vi "Round_Three_Decimals.vi"(11 "Number Input":dbl) -> (3 "Number Output":dbl)   [LabVIEW 2020]
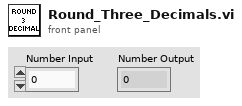
[diagram p1: front panel]
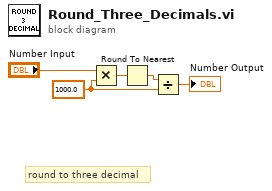
[diagram p0: block diagram]
diagram:
  w1 = 1000.0 ("y")
  # "round to three decimal"
  n1 = Multiply(x="Number Input", y=w1) -> (x*y=w3:dbl)
  n2 = Round To Nearest(number=w3) -> (nearest integer value=w2:dbl)
  n3 = Divide(x=w2, y=w1) -> (x/y=→"Number Output":dbl)
